vi "FPGA_TwoAxisEncoder_revised.vi"() -> ()   [LabVIEW 2015]
uses:
  <vilib>/LabVIEW Targets/FPGA/cRIO/shared/nicrio_ModuleControls/nicrio_cRIO-9361_DecodingType.ctl
  <vilib>/LabVIEW Targets/FPGA/cRIO/shared/nicrio_ModuleControls/nicrio_cRIO-9361_Terminal.ctl
  <vilib>/LabVIEW Targets/FPGA/cRIO/shared/nicrio_ModuleControls/nicrio_cRIO-9361_ZIndexPhase.ctl
  NI 9361 Support Files.llb/NI 9361 Front End DI Reference.ctl
  NI 9361 Support Files.llb/NI 9361 Front End Configuration Array.ctl
  <vilib>/LabVIEW Targets/FPGA/cRIO/shared/nicrio_ModuleControls/nicrio_cRIO-9361_TerminalMode.ctl
  <vilib>/rvi/Emulation/niFpgaGetClockAttributes.vi
  <vilib>/rvi/Emulation/niFpgaSctlEmulationGetInTimedLoop.vi
  <vilib>/rvi/Emulation/niFpgaEmulationReportErrorSimple.vi
  <vilib>/rvi/Emulation/niFpgaCriticalErrorInLSC.vi
  <vilib>/rvi/Emulation/niFpgaProcessEmulError.vi
  <vilib>/rvi/eio/common/nirviEmuTemplateMethod_errors.vi
  <vilib>/rvi/eio/common/nirviEmuTemplatePropertySet_errors.vi
  <vilib>/eio/EIONode/EIONode.xnode
  <vilib>/eio/EIOMethodNode/EIOMethodNode.xnode
  <vilib>/eio/EIOPropertyNode/EIOPropertyNode.xnode
  <vilib>/LabVIEW Targets/FPGA/cRIO/shared/nicrio_ModuleControls/nicrio_cRIO-9361_CounterData.ctl
  <vilib>/LabVIEW Targets/FPGA/cRIO/shared/nicrio_ModuleControls/nicrio_cRIO-9361_CounterStatus.ctl
  <vilib>/rvi/eio/common/nirviEmuTemplatePropertyGet_errors.vi
  <vilib>/rvi/eio/common/nirviEmuTemplatePropertyGet_noerrors.vi
  <vilib>/rvi/eio/common/nirviEmuTemplatePropertySet_noerrors.vi
panel:
  out "Mod5/AI4-XMod2":fxp<+/-,16,5>
  out "Mod5/AI3-XMod1":fxp<+/-,16,5>
  out "Mod5/AI1-ZMod2":fxp<+/-,16,5>
  out "Mod5/AI0-ZMod1(vol)":fxp<+/-,16,5>
  in  "Initial":bool
  out "Line Scale X (count)":i32
  out "Encoder X (count)":i32
  in  "Velocity Command X (vol)":fxp<+/-,20,5>
  out "Output X (vol)":fxp<+/-,20,5>
  out "Line Scale Z (count)":i32
  out "Output Z (vol)":fxp<+/-,20,5>
  in  "Start":bool
  out "Error Out (ENC)":errorcluster
  out "ENC2":bool
  out "ENC1":bool
  out "ENC Ready":bool
  out "DIO Ready":bool
  out "V Loop":bool
  out "Error Out":errorcluster
  in  "Velocity Command Z (vol)":fxp<+/-,20,5>
  in  "Output Votage Bound (vol)":fxp<+,20,5>=1.0
  in  "stop":bool
  out "Encoder Z (count)":i32
  in  "Loop Delay (Tick)":u32=40000
  in  "HOST READY?":bool
  out "SYSTEM INITIALIZED":bool
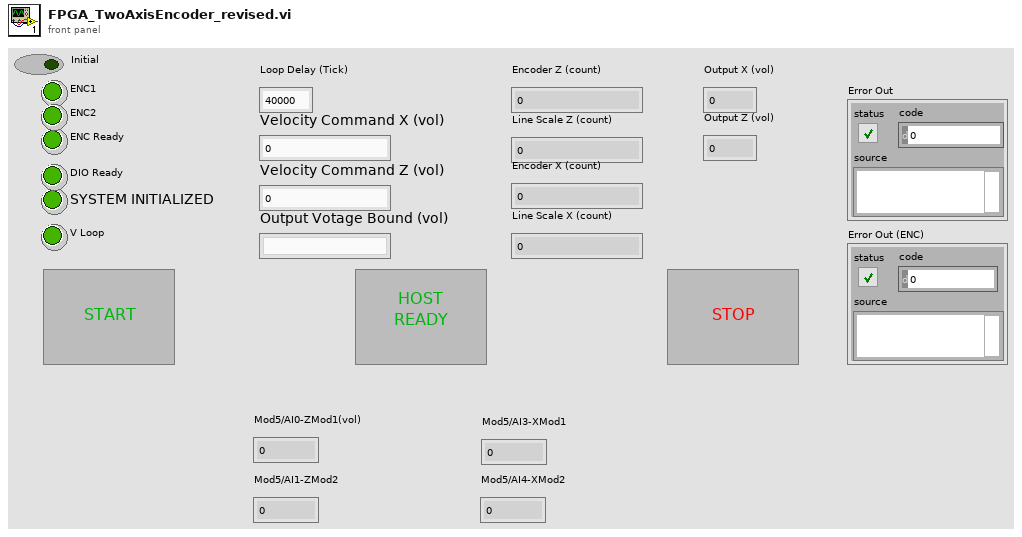
[diagram p1: front panel]
types:
  T1 = typedef "nicrio_cRIO-9361_DecodingType.ctl" = enum8{"x1", "x2", "x4"}
  T2 = typedef "nicrio_cRIO-9361_Terminal.ctl" = enum8{"DI0", "DI1", "DI2", "DI3", "DI4", "DI5", "DI6", "DI7"}
  T3 = typedef "NI 9361 Front End Configuration Array.ctl" = cluster{"Digital Filter Enable":bool, "Digital Filter Minimum Pulse Width":u16, "Terminal Mode":T4}[]
  T4 = typedef "nicrio_cRIO-9361_TerminalMode.ctl" = enum8{"Differential", "Single-Ended", "Single-Ended with Pull-up"}
  T5 = typedef "NI 9361 Front End DI Reference.ctl" = cluster{"DI0":refnum<k21>, "DI1":refnum<k21>, "DI2":refnum<k21>, "DI4":refnum<k21>, "DI5":refnum<k21>, "DI6":refnum<k21>, "DI3":refnum<k21>, "DI7":refnum<k21>}
  T6 = typedef "nicrio_cRIO-9361_ZIndexPhase.ctl" = u8
  T7 = typedef "nicrio_cRIO-9361_CounterData.ctl" = cluster{"A":u32, "B":u32, "Status":T8}
  T8 = typedef "nicrio_cRIO-9361_CounterStatus.ctl" = enum8{"No Sample", "New", "Repeated", "Timeout", "New and Missed", "Timeout and Missed"}
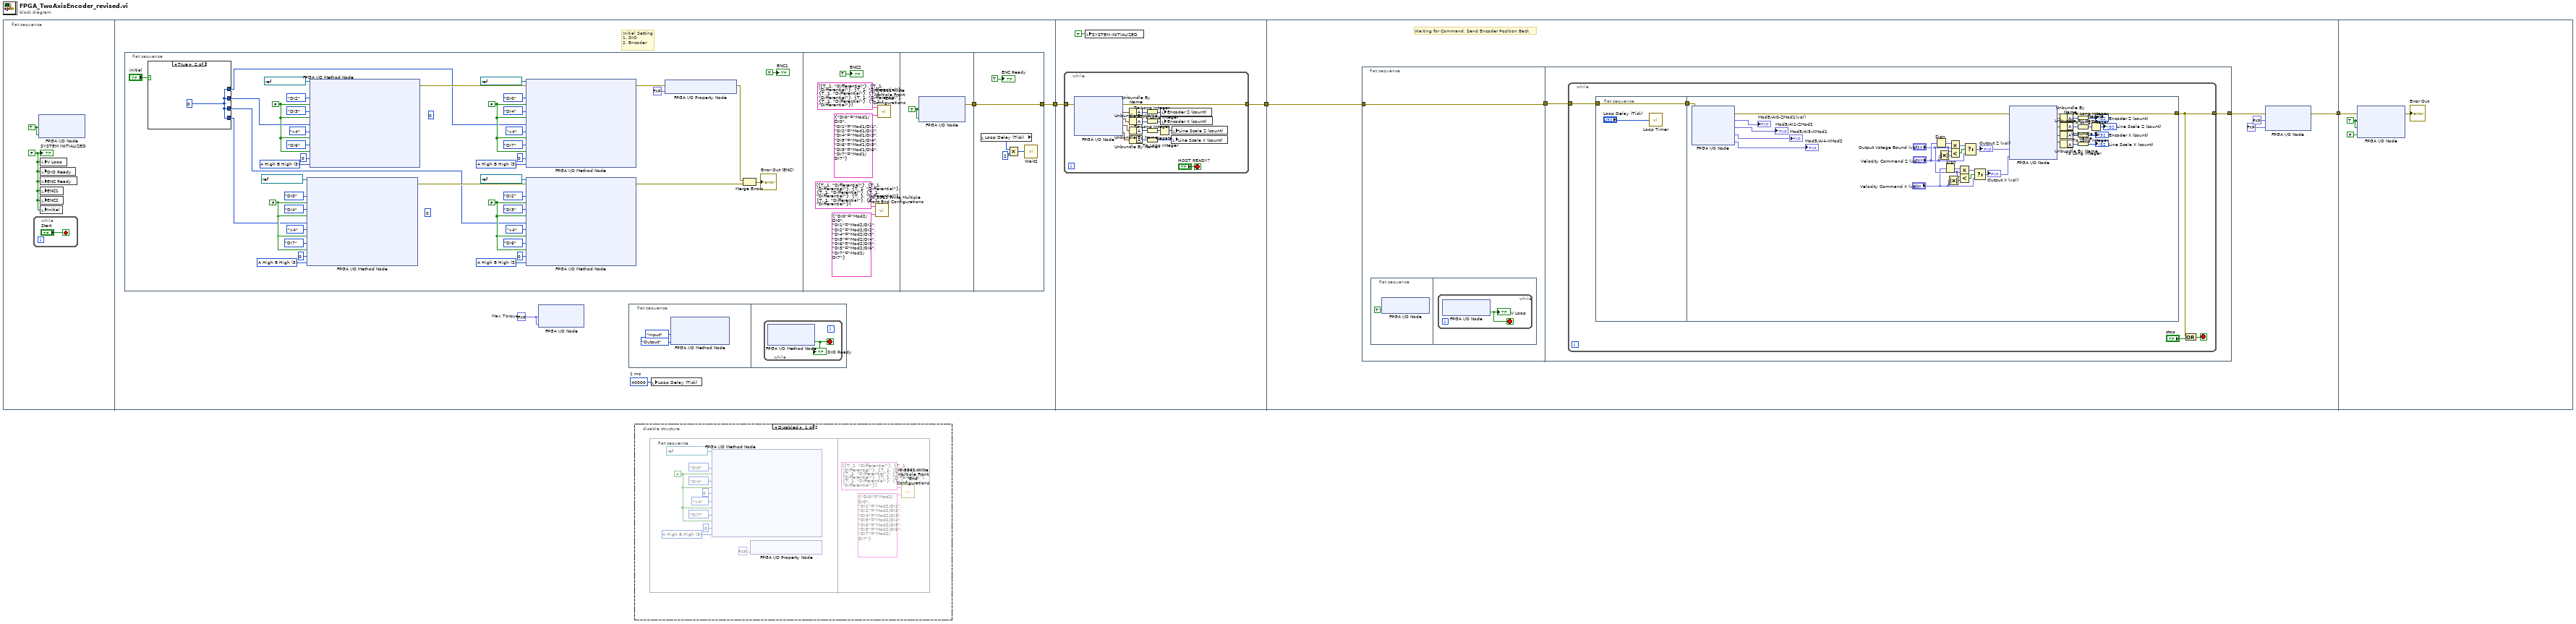
[diagram p0: block diagram]
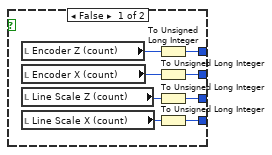
[diagram p3: hidden frame]
diagram:
  n1 = flat-sequence {
    tunnel: [w9] -> w1
    tunnel: [w80] -> w2
    tunnel: w1 -> [w81]
    tunnel: [w101] -> w3
    tunnel: w2 -> [w103]
    tunnel: w3 -> [w153]
    frame #0 {
      w5 = TRUE ("Mod1/Stop")
      w4 = FALSE
      n2 = while {
        stop <- "Start" stop-if-true
      }
      n3 = xnode "FPGA I/O Node"("Mod1/Stop"=w5, "Mod2/Stop"=w5) -> ()  [unwired: 2 in, 2 out]
      n4 = local write "V Loop"(w4) -> ()
      n5 = local write "DIO Ready"(w4) -> ()
      n6 = local write "ENC Ready"(w4) -> ()
      n7 = local write "ENC1"(w4) -> ()
      n8 = local write "ENC2"(w4) -> ()
      n9 = local write "Initial"(w4) -> ()
      "SYSTEM INITIALIZED" <- w4
    }
    frame #1 {
      w7 = fxp<+/-,20,5> 10.0  # Max Torque
      w10 = u32 40000  # 1 ms
      # "Initial Setting\n1. DIO\n2. Encoder"
      n10 = flat-sequence {
        tunnel: [w70] -> w8
        tunnel: [w76] -> w9
        tunnel: w8 -> [w76]
        frame #0 {
          w18 = T6 3 items=["A High B High"=3, "A High B Low"=2, "A Low B High"=1, "A Low B Low"=0] ("Z Index Phase")
          w20 = FALSE
          w27 = T6 3 items=["A High B High"=3, "A High B Low"=2, "A Low B High"=1, "A Low B Low"=0] ("Z Index Phase")
          w29 = FALSE
          (unwired) u32 0 ("Initial Position")
          w38 = T6 3 items=["A High B High"=3, "A High B Low"=2, "A Low B High"=1, "A Low B Low"=0] ("Z Index Phase")
          w40 = FALSE
          (unwired) u32 0 ("Initial Position")
          w49 = T6 3 items=["A High B High"=3, "A High B Low"=2, "A Low B High"=1, "A Low B Low"=0] ("Z Index Phase")
          w51 = FALSE
          n11 = case shown="True" "Initial" {
            tunnel: [w59 w64] -> w11
            tunnel: [w58 w64] -> w12
            tunnel: [w57 w64] -> w13
            tunnel: [w56 w64] -> w14
            frame False {
              n12 = local read "Encoder Z (count)"() -> (w61:i32)
              n13 = local read "Encoder X (count)"() -> (w62:i32)
              n14 = local read "Line Scale Z (count)"() -> (w60:i32)
              n15 = local read "Line Scale X (count)"() -> (w63:i32)
              n16 = To Unsigned Long Integer(number=w61) -> (unsigned 32bit integer=w59:u32)
              n17 = To Unsigned Long Integer(number=w62) -> (unsigned 32bit integer=w58:u32)
              n18 = To Unsigned Long Integer(number=w60) -> (unsigned 32bit integer=w57:u32)
              n19 = To Unsigned Long Integer(number=w63) -> (unsigned 32bit integer=w56:u32)
            }
            frame True {
              w64 = u32 0 ("Initial Position")
            }
          }
          n20 = xnode "FPGA I/O Method Node"("FPGA I/O In"=refnum<k21> "Mod2/CTR1" ("FPGA I/O"), "A Terminal"=nicrio_cRIO-9361_Terminal."DI0", "A Invert Polarity"=w20, "B Terminal"=nicrio_cRIO-9361_Terminal."DI4", "B Invert Polarity"=w20, "Initial Position"=w14, "Decoding Type"=nicrio_cRIO-9361_DecodingType."x4", "Z Index Enable"=w20, "Z Terminal"=nicrio_cRIO-9361_Terminal."DI7", "Z Invert Polarity"=w20, "Z Index Value"=u32 0, "Z Index Phase"=w18) -> ("error out"=w16:errorcluster)  [unwired: 1 in, 1 out]
          n21 = xnode "FPGA I/O Method Node"("FPGA I/O In"=refnum<k21> "Mod1/CTR1" ("FPGA I/O"), "A Terminal"=nicrio_cRIO-9361_Terminal."DI2", "A Invert Polarity"=w29, "B Terminal"=nicrio_cRIO-9361_Terminal."DI3", "B Invert Polarity"=w29, "Initial Position"=w12, "Decoding Type"=nicrio_cRIO-9361_DecodingType."x4", "Z Index Enable"=w29, "Z Terminal"=nicrio_cRIO-9361_Terminal."DI6", "Z Invert Polarity"=w29, "Z Index Value"=u32 0, "Z Index Phase"=w27) -> ("error out"=w25:errorcluster)  [unwired: 1 in, 1 out]
          n22 = xnode "FPGA I/O Method Node"("error in"=w25, "FPGA I/O In"=refnum<k21> "Mod1/CTR0" ("FPGA I/O"), "A Terminal"=nicrio_cRIO-9361_Terminal."DI0", "A Invert Polarity"=w51, "B Terminal"=nicrio_cRIO-9361_Terminal."DI4", "B Invert Polarity"=w51, "Initial Position"=w11, "Decoding Type"=nicrio_cRIO-9361_DecodingType."x4", "Z Index Enable"=w51, "Z Terminal"=nicrio_cRIO-9361_Terminal."DI7", "Z Invert Polarity"=w51, "Z Index Value"=u32 0, "Z Index Phase"=w49) -> ("error out"=w45:errorcluster)  [unwired: 1 out]
          n23 = xnode "FPGA I/O Method Node"("error in"=w16, "FPGA I/O In"=refnum<k21> "Mod2/CTR0" ("FPGA I/O"), "A Terminal"=nicrio_cRIO-9361_Terminal."DI2", "A Invert Polarity"=w40, "B Terminal"=nicrio_cRIO-9361_Terminal."DI3", "B Invert Polarity"=w40, "Initial Position"=w13, "Decoding Type"=nicrio_cRIO-9361_DecodingType."x4", "Z Index Enable"=w40, "Z Terminal"=nicrio_cRIO-9361_Terminal."DI6", "Z Invert Polarity"=w40, "Z Index Value"=u32 0, "Z Index Phase"=w38) -> ("error out"=w36:errorcluster)  [unwired: 1 out]
          n24 = xnode "FPGA I/O Property Node"("error in"=w45, "Digital Logic Threshold"=fxp<+/-,16,5> 2.0) -> ("error out"=w35:errorcluster)  [unwired: 1 in, 1 out]
          n25 = Merge Errors(w35, w36) -> (→"Error Out (ENC)":errorcluster)
          "ENC1" <- TRUE ("ENC1")
        }
        frame #1 {
          n26 = call "NI 9361 Write Multiple Front End Configurations.vi"("FPGA Front End DI"=T5 {"DI0"="Mod2/DI0", "DI1"="Mod2/DI1", "DI2"="Mod2/DI2", "DI4"="Mod2/DI3", "DI5"="Mod2/DI4", "DI6"="Mod2/DI5", "DI3"="Mod2/DI6", "DI7"="Mod2/DI7"}, "Front End Configuration"=T3 [{"Digital Filter Enable"=TRUE, "Digital Filter Minimum Pulse Width"=1, "Terminal Mode"=enum."Differential"}, {"Digital Filter Enable"=TRUE, "Digital Filter Minimum Pulse Width"=1, "Terminal Mode"=enum."Differential"}, {"Digital Filter Enable"=TRUE, "Digital Filter Minimum Pulse Width"=1, "Terminal Mode"=enum."Differential"}, {"Digital Filter Enable"=TRUE, "Digital Filter Minimum Pulse Width"=1, "Terminal Mode"=enum."Differential"}, {"Digital Filter Enable"=TRUE, "Digital Filter Minimum Pulse Width"=1, "Terminal Mode"=enum."Differential"}, {"Digital Filter Enable"=TRUE, "Digital Filter Minimum Pulse Width"=1, "Terminal Mode"=enum."Differential"}, {"Digital Filter Enable"=TRUE, "Digital Filter Minimum Pulse Width"=1, "Terminal Mode"=enum."Differential"}, {"Digital Filter Enable"=TRUE, "Digital Filter Minimum Pulse Width"=1, "Terminal Mode"=enum."Differential"}]) -> ()  [unwired: 1 in]
          n27 = call "NI 9361 Write Multiple Front End Configurations.vi"("FPGA Front End DI"=T5 {"DI0"="Mod1/DI0", "DI1"="Mod1/DI1", "DI2"="Mod1/DI2", "DI4"="Mod1/DI3", "DI5"="Mod1/DI4", "DI6"="Mod1/DI5", "DI3"="Mod1/DI6", "DI7"="Mod1/DI7"}, "Front End Configuration"=T3 [{"Digital Filter Enable"=TRUE, "Digital Filter Minimum Pulse Width"=1, "Terminal Mode"=enum."Differential"}, {"Digital Filter Enable"=TRUE, "Digital Filter Minimum Pulse Width"=1, "Terminal Mode"=enum."Differential"}, {"Digital Filter Enable"=TRUE, "Digital Filter Minimum Pulse Width"=1, "Terminal Mode"=enum."Differential"}, {"Digital Filter Enable"=TRUE, "Digital Filter Minimum Pulse Width"=1, "Terminal Mode"=enum."Differential"}, {"Digital Filter Enable"=TRUE, "Digital Filter Minimum Pulse Width"=1, "Terminal Mode"=enum."Differential"}, {"Digital Filter Enable"=TRUE, "Digital Filter Minimum Pulse Width"=1, "Terminal Mode"=enum."Differential"}, {"Digital Filter Enable"=TRUE, "Digital Filter Minimum Pulse Width"=1, "Terminal Mode"=enum."Differential"}, {"Digital Filter Enable"=TRUE, "Digital Filter Minimum Pulse Width"=1, "Terminal Mode"=enum."Differential"}]) -> ()  [unwired: 1 in]
          "ENC2" <- TRUE ("ENC2")
        }
        frame #2 {
          w71 = TRUE ("Mod1/Start")
          n28 = xnode "FPGA I/O Node"("Mod1/Start"=w71, "Mod2/Start"=w71) -> ("error out"=w70:errorcluster)  [unwired: 3 in, 2 out]
        }
        frame #3 {
          n29 = local read "Loop Delay (Tick)"() -> (w73:u32)
          n30 = Multiply(x=w73, y=u32 2) -> (x*y=w72:u32)
          n31 = call "Wait2"("Count(Ticks)"=w72) -> ()  [unwired: 1 out]
          "ENC Ready" <- TRUE ("ENC Ready")
        }
      }
      n32 = xnode "FPGA I/O Node"("Mod3/AO1"=w7, "Mod3/AO3"=w7) -> ()  [unwired: 2 in, 2 out]
      n33 = flat-sequence {
        frame #0 {
          n34 = xnode "FPGA I/O Method Node"("DIO 7:4"=enum8{"No Change", "Input", "Output"}."Input", "DIO 3:0"=enum8{"No Change", "Input", "Output"}."Output" ("DIO 7:4")) -> ()  [unwired: 1 in, 1 out]
        }
        frame #1 {
          n35 = while {
            stop <- w79 stop-if-true
            n36 = xnode "FPGA I/O Method Node"() -> ("Ready"=w79:bool)  [unwired: 1 in, 1 out]
            "DIO Ready" <- w79
          }
        }
      }
      n37 = local write "Loop Delay (Tick)"(w10) -> ()
    }
    frame #2 {
      n38 = while {
        tunnel: w81 -> [w97]
        tunnel: [w96] -> w80
        stop <- "HOST READY?" stop-if-true
        n39 = xnode "FPGA I/O Node"("error in"=w97) -> ("error out"=w96:errorcluster, "Mod1/CTR0"=w91:T7, "Mod1/CTR1"=w90:T7, "Mod2/CTR0"=w84:T7, "Mod2/CTR1"=w83:T7)  [unwired: 4 in, 4 out]
        n40 = Unbundle By Name(w91) -> ("A"=w92:u32)
        n41 = Unbundle By Name(w90) -> ("A"=w93:u32)
        n42 = Unbundle By Name(w84) -> ("A"=w89:u32)
        n43 = Unbundle By Name(w83) -> ("A"=w86:u32)
        n44 = To Long Integer(number=w92) -> (32bit integer=w94:i32)
        n45 = To Long Integer(number=w93) -> (32bit integer=w95:i32)
        n46 = To Long Integer(number=w89) -> (32bit integer=w88:i32)
        n47 = To Long Integer(number=w86) -> (32bit integer=w85:i32)
        n48 = Negate(x=w88) -> (-x=w87:i32)
        n49 = local write "Encoder Z (count)"(w94) -> ()
        n50 = local write "Encoder X (count)"(w95) -> ()
        n51 = local write "Line Scale X (count)"(w85) -> ()
        n52 = local write "Line Scale Z (count)"(w87) -> ()
      }
      n53 = local write "SYSTEM INITIALIZED"(TRUE ("SYSTEM INITIALIZED")) -> ()
    }
    frame #3 {
      # "Waiting for Command, Send Encoder Position Back"
      n54 = flat-sequence {
        tunnel: w103 -> [w105]
        tunnel: [w105] -> w104
        tunnel: w104 -> [w109]
        tunnel: [w108] -> w102
        frame #0 {
          n55 = flat-sequence {
            frame #0 {
              n56 = xnode "FPGA I/O Node"("Mod4/DIO0"=TRUE) -> ()  [unwired: 1 in, 1 out]
            }
            frame #1 {
              n57 = while {
                stop <- w107 stop-if-true
                n58 = xnode "FPGA I/O Node"() -> ("Mod4/DIO4"=w107:bool)  [unwired: 1 in, 1 out]
                "V Loop" <- w107
              }
            }
          }
        }
        frame #1 {
          n59 = while {
            tunnel: w109 -> [w113]
            tunnel: [w111] -> w108
            stop <- w112 stop-if-true
            n60 = flat-sequence {
              tunnel: w113 -> [w116]
              tunnel: [w116] -> w114
              tunnel: w114 -> [w122]
              tunnel: [w147] -> w111
              frame #0 {
                n61 = call "Loop Timer"("Count(Ticks)"="Loop Delay (Tick)") -> ()  [unwired: 1 out]
              }
              frame #1 {
                n62 = xnode "FPGA I/O Node"("error in"=w122) -> ("error out"=w121:errorcluster, "Mod5/AI0"=→"Mod5/AI0-ZMod1(vol)":fxp<+/-,16,5>, "Mod5/AI1"=→"Mod5/AI1-ZMod2":fxp<+/-,16,5>, "Mod5/AI3"=→"Mod5/AI3-XMod1":fxp<+/-,16,5>, "Mod5/AI4"=→"Mod5/AI4-XMod2":fxp<+/-,16,5>)  [unwired: 4 in, 4 out]
                n63 = Sign(1:"Velocity Command Z (vol)") -> (0:w143:fxp<+/-,2,2>)
                n64 = Absolute Value(x="Velocity Command Z (vol)") -> (abs(x)=w142:fxp<+,20,5>)
                n65 = Sign(1:"Velocity Command X (vol)") -> (0:w137:fxp<+/-,2,2>)
                n66 = Absolute Value(x="Velocity Command X (vol)") -> (abs(x)=w136:fxp<+,20,5>)
                n67 = Multiply(x=w143, y="Output Votage Bound (vol)") -> (x*y=w144:fxp<+/-,20,5>)
                n68 = Less?(x="Output Votage Bound (vol)", y=w142) -> (x < y?=w141:bool)
                n69 = Multiply(x=w137, y="Output Votage Bound (vol)") -> (x*y=w138:fxp<+/-,20,5>)
                n70 = Less?(x="Output Votage Bound (vol)", y=w136) -> (x < y?=w135:bool)
                n71 = Select(t=w144, s=w141, f="Velocity Command Z (vol)") -> (s? t:f=w131:fxp<+/-,20,5>)
                "Output Z (vol)" <- w131
                n72 = Select(t=w138, s=w135, f="Velocity Command X (vol)") -> (s? t:f=w132:fxp<+/-,20,5>)
                "Output X (vol)" <- w132
                n73 = xnode "FPGA I/O Node"("error in"=w121, "Mod3/AO0"=w131, "Mod3/AO2"=w132) -> ("error out"=w147:errorcluster, "Mod1/CTR0"=w149:T7, "Mod2/CTR0"=w139:T7, "Mod1/CTR1"=w126:T7, "Mod2/CTR1"=w125:T7)  [unwired: 6 in, 6 out]
                n74 = Unbundle By Name(w149) -> ("A"=w148:u32)
                n75 = Unbundle By Name(w139) -> ("A"=w146:u32)
                n76 = Unbundle By Name(w126) -> ("A"=w130:u32)
                n77 = Unbundle By Name(w125) -> ("A"=w129:u32)
                n78 = To Long Integer(number=w148) -> (32bit integer=→"Encoder Z (count)":i32)
                n79 = To Long Integer(number=w146) -> (32bit integer=w124:i32)
                n80 = To Long Integer(number=w130) -> (32bit integer=→"Encoder X (count)":i32)
                n81 = To Long Integer(number=w129) -> (32bit integer=→"Line Scale X (count)":i32)
                n82 = Negate(x=w124) -> (-x=→"Line Scale Z (count)":i32)
              }
            }
            n83 = Compound Arithmetic op=OR(w111, "stop") -> (w112:bool)
          }
        }
      }
      n84 = xnode "FPGA I/O Node"("error in"=w102, "Mod3/AO0"=fxp<+/-,20,5> 0.0, "Mod3/AO2"=fxp<+/-,20,5> 0.0) -> ("error out"=w101:errorcluster)  [unwired: 2 in, 2 out]
    }
    frame #4 {
      w151 = TRUE ("Mod1/Stop")
      n85 = xnode "FPGA I/O Node"("error in"=w153, "Mod1/Stop"=w151, "Mod2/Stop"=w151, "Mod4/DIO0"=FALSE) -> ("error out"=→"Error Out":errorcluster)  [unwired: 3 in, 3 out]
    }
  }
  n86 = disable-structure shown="Disabled" {
    frame Disabled {
      n87 = flat-sequence {
        frame #0 {
          w157 = T6 3 items=["A High B High"=3, "A High B Low"=2, "A Low B High"=1, "A Low B Low"=0] ("Z Index Phase")
          w159 = FALSE
          n88 = xnode "FPGA I/O Method Node"("FPGA I/O In"=refnum<k21> "Mod2/CTR0" ("FPGA I/O"), "A Terminal"=nicrio_cRIO-9361_Terminal."DI0", "A Invert Polarity"=w159, "B Terminal"=nicrio_cRIO-9361_Terminal."DI4", "B Invert Polarity"=w159, "Initial Position"=u32 0, "Decoding Type"=nicrio_cRIO-9361_DecodingType."x4", "Z Index Enable"=w159, "Z Terminal"=nicrio_cRIO-9361_Terminal."DI7", "Z Invert Polarity"=w159, "Z Index Value"=u32 0, "Z Index Phase"=w157) -> ()  [unwired: 1 out]
          n89 = xnode "FPGA I/O Property Node"("Digital Logic Threshold"=fxp<+/-,16,5> 2.0) -> ()  [unwired: 1 in, 1 out]
        }
        frame #1 {
          n90 = call "NI 9361 Write Multiple Front End Configurations.vi"("FPGA Front End DI"=T5 {"DI0"="Mod2/DI0", "DI1"="Mod2/DI1", "DI2"="Mod2/DI2", "DI4"="Mod2/DI3", "DI5"="Mod2/DI4", "DI6"="Mod2/DI5", "DI3"="Mod2/DI6", "DI7"="Mod2/DI7"}, "Front End Configuration"=T3 [{"Digital Filter Enable"=TRUE, "Digital Filter Minimum Pulse Width"=1, "Terminal Mode"=enum."Differential"}, {"Digital Filter Enable"=TRUE, "Digital Filter Minimum Pulse Width"=1, "Terminal Mode"=enum."Differential"}, {"Digital Filter Enable"=TRUE, "Digital Filter Minimum Pulse Width"=1, "Terminal Mode"=enum."Differential"}, {"Digital Filter Enable"=TRUE, "Digital Filter Minimum Pulse Width"=1, "Terminal Mode"=enum."Differential"}, {"Digital Filter Enable"=TRUE, "Digital Filter Minimum Pulse Width"=1, "Terminal Mode"=enum."Differential"}, {"Digital Filter Enable"=TRUE, "Digital Filter Minimum Pulse Width"=1, "Terminal Mode"=enum."Differential"}, {"Digital Filter Enable"=TRUE, "Digital Filter Minimum Pulse Width"=1, "Terminal Mode"=enum."Differential"}, {"Digital Filter Enable"=TRUE, "Digital Filter Minimum Pulse Width"=1, "Terminal Mode"=enum."Differential"}]) -> ()  [unwired: 1 in]
        }
      }
    }
    frame Enabled {
    }
  }
